vi "Initialize.vi"(9 "State Variables in":T1={"NIVS.CachedDataRef"=refnum, "NIVS.LaunchRef"=refnum, "NIVS.SysDefRoot"=refnum, "NIVS.Workspace"=refnum, "NIVS.CachedData"={"Name"="", "Node Path"="", "Caption"="", "List"={"AutoUpdate"=FALSE, "Names"=[], "Values"=[], "Symbols"=[]}}, "NIVS.SystemStateRefs"={"CustDatRef"=refnum, "EvtRef"=refnum, "Target State User Event"=refnum}, "NIVS.UserEventRefs"={"SystemChangeEventRef"=refnum, "Event Registration Refnum"=refnum}, "Workspace.Connected?"=FALSE, "Workspace.ChannelFound?"=FALSE, "UI.Listbox"=refnum, "VS.DisplayFilter"=7, "Force?"=FALSE} {"VS.DisplayFilter" items=["K_CHAN_R", "K_CHAN_W", "K_CHAN_RW", "K_CHAN_VOLT", "K_CHAN_FAULT", "K_ALL", "K_CUSTOM", "K_CHAN_R_VIS", "K_CHAN_W_VIS", "K_CHAN_RW_VIS", "K_CHAN_VOLT_VIS", "K_CHAN_FAULT_VIS"]}, 10 "Item.Data":T7, 11 "NIVS.Gateway IP Address":string) -> (0 "error out":errorcluster, 3 "State Variables in":T1={"NIVS.CachedDataRef"=refnum, "NIVS.LaunchRef"=refnum, "NIVS.SysDefRoot"=refnum, "NIVS.Workspace"=refnum, "NIVS.CachedData"={"Name"="", "Node Path"="", "Caption"="", "List"={"AutoUpdate"=FALSE, "Names"=[], "Values"=[], "Symbols"=[]}}, "NIVS.SystemStateRefs"={"CustDatRef"=refnum, "EvtRef"=refnum, "Target State User Event"=refnum}, "NIVS.UserEventRefs"={"SystemChangeEventRef"=refnum, "Event Registration Refnum"=refnum}, "Workspace.Connected?"=FALSE, "Workspace.ChannelFound?"=FALSE, "UI.Listbox"=refnum, "VS.DisplayFilter"=7, "Force?"=FALSE} {"VS.DisplayFilter" items=["K_CHAN_R", "K_CHAN_W", "K_CHAN_RW", "K_CHAN_VOLT", "K_CHAN_FAULT", "K_ALL", "K_CUSTOM", "K_CHAN_R_VIS", "K_CHAN_W_VIS", "K_CHAN_RW_VIS", "K_CHAN_VOLT_VIS", "K_CHAN_FAULT_VIS"]})   [LabVIEW 2015, in "Workspace.Obejct.Radio.lvlib"]
uses:
  Workspace.Obejct.Radio.lvlib
  Types/StateVariables.ctl
  <vilib>/NI Veristand/Display Template Support/Display Template Support.llb/enum_Display Template Handler Minimal To Workspace.ctl
  <vilib>/NI Veristand/Display Template Support/Display Template Support.llb/enum_Display Template Handler Minimal To Widget Msg.ctl
  NationalInstruments.VeriStand.SystemStorage
  <vilib>/NI Veristand/Execution/Workspace/WorkspaceAPI.ctl
  NationalInstruments.VeriStand.ClientAPI
  Types/SavedStateData.ctl
  Types/Config.ctl
  <vilib>/NI Veristand/Execution/Workspace/SystemStateEventRef.ctl
  <vilib>/NI Veristand/Execution/Workspace/Target State Info.ctl
  <vilib>/NI Veristand/Execution/Workspace/Target State.ctl
  <vilib>/NI Veristand/Execution/Workspace/SystemStateRegEventRef.ctl
  <vilib>/NI Veristand/Display Template Support/Display Template Support.llb/cluster_Screen Item Settings.ctl
  <vilib>/NI Veristand/Display Template Support/Display Template Support.llb/cluster_Graph Scale Settings.ctl
  <vilib>/NI Veristand/Display Template Support/Display Template Support.llb/cluster_Graph Plot Settings.ctl
  <vilib>/NI Veristand/Execution/Workspace/NI_VS Workspace ExecutionAPI.lvlib
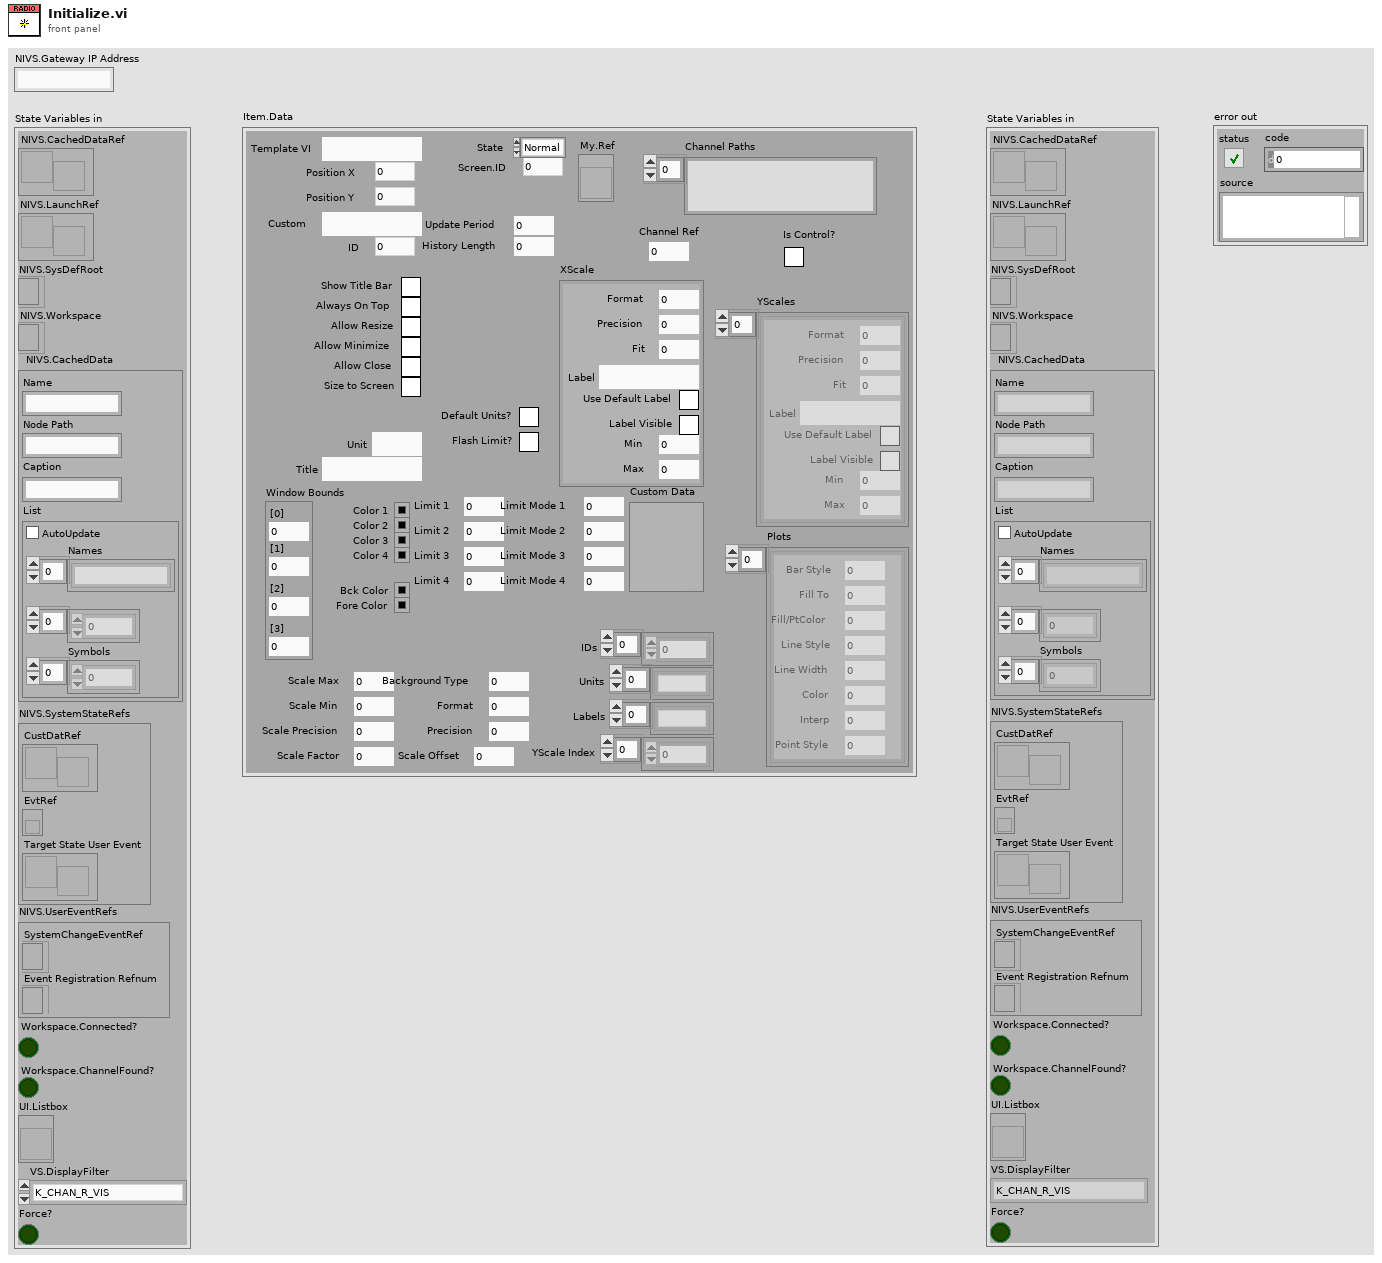
[diagram p1: front panel]
types:
  T1 = typedef "Workspace.Obejct.Radio.lvlib/StateVariables.ctl" = cluster{"NIVS.CachedDataRef":refnum<user-event>, "NIVS.LaunchRef":refnum<user-event>, "NIVS.SysDefRoot":refnum<k24>, "NIVS.Workspace":T2, "NIVS.CachedData":T3, "NIVS.SystemStateRefs":T5, "NIVS.UserEventRefs":cluster{"SystemChangeEventRef":T6, "Event Registration Refnum":refnum<event-registration>}, "Workspace.Connected?":bool, "Workspace.ChannelFound?":bool, "UI.Listbox":refnum<vi>, "VS.DisplayFilter":u8, "Force?":bool}
  T2 = typedef "NI_VS Workspace ExecutionAPI.lvlib/WorkspaceAPI.ctl" = refnum<k24>
  T3 = typedef "Workspace.Obejct.Radio.lvlib/SavedStateData.ctl" = cluster{"Name":string, "Node Path":string, "Caption":string, "List":T4}
  T4 = typedef "Workspace.Obejct.Radio.lvlib/Config.ctl" = cluster{"AutoUpdate":bool, "Names":string[], "Values":dbl[], "Symbols":i32[]}
  T5 = typedef "NI_VS Workspace ExecutionAPI.lvlib/SystemStateEventRef.ctl" = cluster{"CustDatRef":refnum<user-event>, "EvtRef":refnum<k27>, "Target State User Event":refnum<user-event>}
  T6 = typedef "NI_VS Workspace ExecutionAPI.lvlib/SystemStateRegEventRef.ctl" = refnum<event-registration>
  T7 = typedef "cluster_Screen Item Settings.ctl" = cluster{"Template VI":string, "Position X":i32, "Position Y":i32, "Custom":string, "Show Title Bar":bool, "ID":i32, "Always On Top":bool, "Allow Resize":bool, "Allow Minimize":bool, "Allow Close":bool, "Size to Screen":bool, "Screen.ID":i32, "State":enum16{"Normal", "New"}, "Title":string, "Window Bounds":cluster{"[0]":i16, "[1]":i16, "[2]":i16, "[3]":i16}, "Channel Ref":u64, "Unit":string, "Default Units?":bool, "Flash Limit?":bool, "Color 1":u32, "Color 2":u32, "Color 3":u32, "Color 4":u32, "Bck Color":u32, "Fore Color":u32, "Limit 1":dbl, "Limit 2":dbl, "Limit 3":dbl, "Limit 4":dbl, "Limit Mode 1":i32, "Limit Mode 2":i32, "Limit Mode 3":i32, "Limit Mode 4":i32, "Scale Precision":i32, "Scale Min":dbl, "Scale Max":dbl, "Format":i32, "Precision":i32, "Background Type":i32, "IDs":i32[], "Units":string[], "Labels":string[], "Scale Factor":dbl, "Scale Offset":dbl, "YScale Index":u32[], "XScale":T8, "YScales":T8[], "Plots":T9[], "Update Period":dbl, "History Length":dbl, "My.Ref":refnum<vi>, "Is Control?":bool, "Channel Paths":string[], "Custom Data":variant}
  T8 = typedef "cluster_Graph Scale Settings.ctl" = cluster{"Format":u8, "Precision":u8, "Fit":u8, "Label":string, "Use Default Label":bool, "Label Visible":bool, "Min":dbl, "Max":dbl}
  T9 = typedef "cluster_Graph Plot Settings.ctl" = cluster{"Bar Style":u8, "Fill To":i16, "Fill/PtColor":u32, "Line Style":u8, "Line Width":u8, "Color":u32, "Interp":u8, "Point Style":u8}
  T10 = cluster{"SystemChangeEventRef":T6, "Event Registration Refnum":refnum<event-registration>}
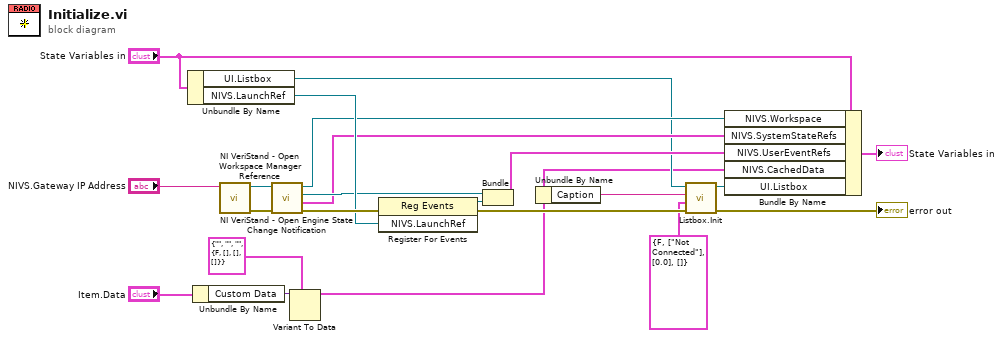
[diagram p0: block diagram]
diagram:
  n1 = Unbundle By Name("State Variables in") -> ("UI.Listbox"=w5:refnum<vi>, "NIVS.LaunchRef"=w15:refnum<user-event>)
  n2 = Unbundle By Name("Item.Data") -> ("Custom Data"=w19:variant)
  n3 = call <vilib>:"NI VeriStand - Open Workspace Manager Reference.vi"("Gateway IP Address (\"\": localhost)"="NIVS.Gateway IP Address") -> ("error out"=w20:errorcluster, "WorkspaceManager"=w21:T2)  [unwired: 9 in]
  n4 = call <vilib>:"NI VeriStand - Open Engine State Change Notification.vi"("error in (no error)"=w20, "WorkspaceManager in"=w21) -> ("error out"=w18:errorcluster, "SystemStateRefs"=w11:T5, "SystemChangeEventRef"=w14:T6, "WorkspaceManager out"=w12:T2)  [unwired: 6 in]
  n5 = Variant To Data(type=T3 {"Name"="", "Node Path"="", "Caption"="", "List"={"AutoUpdate"=FALSE, "Names"=[], "Values"=[], "Symbols"=[]}} ("Cluster"), Variant=w19) -> (data=w3:T3)  [unwired: 1 in, 1 out]
  n6 = register-events(error in=w18, w15) -> (reference out=w22:refnum<event-registration>, error out=w7:errorcluster)  [unwired: 1 in]
  n7 = Bundle("SystemChangeEventRef"=w14, "Event Registration Refnum"=w22) -> (w10:T10)  [unwired: 1 in]
  n8 = Unbundle By Name(w3) -> ("Caption"=w2:string)
  n9 = call "Listbox.Init.vi"("error in (no error)"=w7, "Config"=T4 {"AutoUpdate"=FALSE, "Names"=["Not Connected"], "Values"=[0.0], "Symbols"=[]} ("List"), "Caption.Text"=w2, "Listbox"=w5) -> ("error out"=→"error out":errorcluster, "Listbox"=w4:refnum<vi>)  [unwired: 6 in]
  n10 = Bundle By Name(cluster="State Variables in", "NIVS.Workspace"=w12, "NIVS.SystemStateRefs"=w11, "NIVS.UserEventRefs"=w10, "NIVS.CachedData"=w3, "UI.Listbox"=w4) -> (→"State Variables in":T1)
